vi "Read SA Pin.vi"(8 "error in (no error)":errorcluster, 11 "NR_ACP in":refnum<class "NR_ACP.lvclass">) -> (0 "error out":errorcluster, 2 "SA Pin":string, 3 "NR_ACP out":refnum<class "NR_ACP.lvclass">)   [LabVIEW 2018, in "SeqAuto Evaluations.lvlib" / "NR_ACP.lvclass"]
uses:
  NR_ACP.lvclass
  NR_ACP.lvclass/NR_ACP.ctl
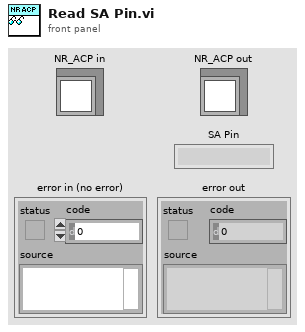
[diagram p1: front panel]
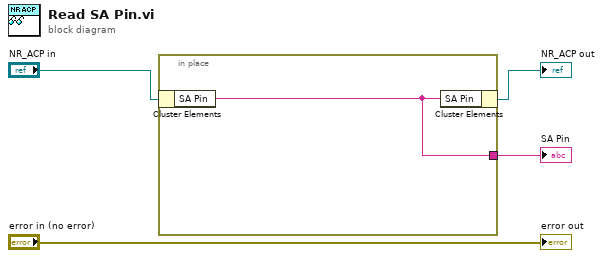
[diagram p0: block diagram]
diagram:
  n1 = in-place {
    in-place-border: [w5] -> w1
    n2 = in-place-cluster #1("NR_ACP in") -> ("SA Pin"=w5:string)
    n3 = in-place-cluster #1("SA Pin"=w5) -> (→"NR_ACP out":refnum<class "NR_ACP.lvclass">)
  }
  "SA Pin" <- w1
  "error out" <- "error in (no error)"
